vi "Check Deviation Attributes.vi"(8 "error in (no error)":errorcluster, 11 "Deviation In":string) -> (0 "error out":errorcluster, 3 "Deviation Out":string)   [LabVIEW 2019, in "Path Settings.lvclass"]
uses:
  Path Settings.lvclass
  subVIs/typedefs/Schedule Types/Schedule--Formula.ctl
  <vilib>/JDP Science/JSONtext/Next JSON Value.vi
  <vilib>/JDP Science/JSONtext/String Subset.vi
  <vilib>/JDP Science/JSONtext/Parsing/Advance past next JSON Value (inlined COPY).vi
  <vilib>/JDP Science/JSONtext/Parsing/Advance past whitespace.vi
  <vilib>/JDP Science/JSONtext/Parsing/Advance past String.vi
  <vilib>/JDP Science/JSONtext/Parsing/Advance past Number.vi
  <vilib>/JDP Science/JSONtext/Parsing/Advance past Line Ending.vi
  <vilib>/JDP Science/JSONtext/Parsing/Parse Full Path or Item Name.vi
  <vilib>/JDP Science/JSONtext/Parsing/Advance past Array.vi
  <vilib>/JDP Science/JSONtext/Parsing/Advance past Object.vi
  <vilib>/JDP Science/JSONtext/support/Error Cluster From Code.vi
  <vilib>/JDP Science/JSONtext/Offset/Find Item Locations by Path.vi
  ObjectSettings/ObjectSettings.lvclass
  <vilib>/JDP Science/JSONtext/JSONtext.lvlib
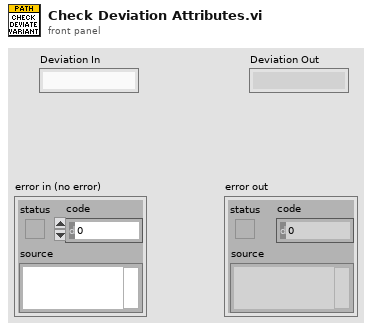
[diagram p1: front panel]
types:
  T1 = typedef "Schedule--Formula.ctl" = cluster{"formula":string, "formula length (nm)":dbl, "formula resolution (nm)":dbl}
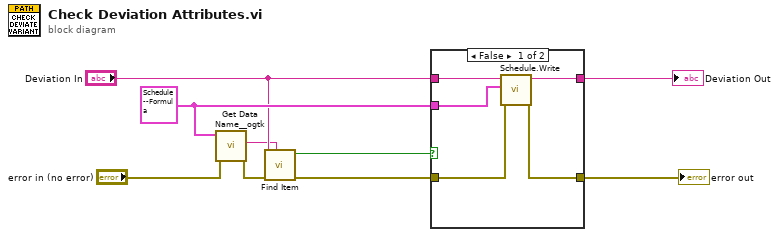
[diagram p0: block diagram]
diagram:
  w9 = T1 {"formula"="1*(step(170-t)*cos(0.62831853071*t)+step(t-170)*cos(0.62831853071*(t-170))*(-1))", "formula length (nm)"=340.0, "formula resolution (nm)"=0.001} ("Formula")
  n1 = call <userlib>:"Get Data Name__ogtk.vi"("error in (no error)"="error in (no error)", "Data"=w9) -> ("error out"=w3:errorcluster, "Data Name"=w1:string)  [unwired: 7 in, 1 out]
  n2 = call <vilib>:"Find Item.vi"("$Path or Item Name"=w1, "error in (no error)"=w3, "JSON"="Deviation In") -> ("error out"=w5:errorcluster, "Found"=w4:bool)  [unwired: 5 in, 2 out]
  n3 = case shown="False" w4 {
    tunnel: w9 -> [w14 _]
    tunnel: "Deviation In" -> [w13 w16]
    tunnel: [w12 w16] -> w6
    tunnel: [w11 w15] -> w7
    tunnel: w5 -> [w10 w15]
    frame False {
      n4 = call "Schedule.Write.vi"("error in (no error)"=w10, "Data to Write"=w14, "Schedule <JSON> In"=w13) -> ("error out"=w11:errorcluster, "Schedule <JSON> Out"=w12:string)  [unwired: 7 in]
    }
    frame True {
    }
  }
  "error out" <- w7
  "Deviation Out" <- w6
